vi "BotSpeak_GetVarVal.vi"(0 "Variable In":string="power") -> (2 "number":dbl)   [LabVIEW 2014]
doc: "Retrieves the value of \"Variable in\" and returns that as \"value\". If the value is a number, this VI also returns that value in double format as \"number\"."
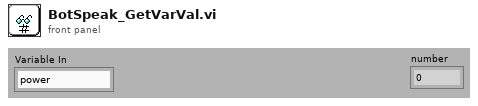
[diagram p1: front panel]
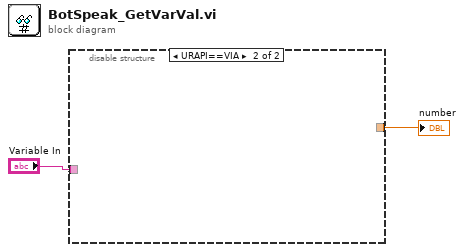
[diagram p0: block diagram]
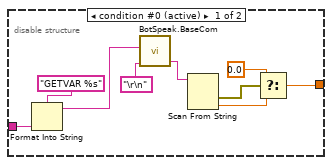
[diagram p2: hidden frame]
diagram:
  n1 = disable-structure shown="URAPI==VIA" {
    disable-tunnel: [w8 _] -> w2
    disable-tunnel: "Variable In" -> [w4 _]
    frame condition #0 (active) {
      n2 = Format Into String(format string="GETVAR %s" ("command"), w4) -> (resulting string=w7:string)  [unwired: 2 in, 1 out]
      n3 = call <userlib>:"BotSpeak.BaseCom.vi"("Termination"="\r\n", "command"=w7) -> ("response"=w3:string)  [unwired: 3 in, 1 out]
      n4 = Scan From String(input string=w3) -> (error out=w11:errorcluster, output 1=w9:dbl)  [unwired: 4 in, 2 out]
      n5 = Select(t=0.0, s=w11, f=w9) -> (s? t:f=w8:dbl)
    }
    frame condition #1 {
    }
  }
  "number" <- w2
